vi "generateSignedDecimalFractions.vi"(6 "timeout (10000)":i32=10000, 8 "error in (no error)":errorcluster, 11 "Parameters":T2={"params"={"apiKey"="", "n"=0, "decimalPlaces"=0, "replacement"=TRUE}, "id"=0.0}) -> (0 "error out":errorcluster, 3 "Response":T1={"result"={"random"={"method"="", "hashedApiKey"="", "n"=0, "decimalPlaces"=0, "replacement"=TRUE, "data"=[], "completionTime"="", "serialNumber"=0}, "signature"="", "bitsUsed"=0, "bitsLeft"=0, "requestsLeft"=0, "advisoryDelay"=0}, "id"=0.0} {"result"."random"."data" format="%#_14g"}, 4 "error data":string[](array[string]))   [LabVIEW 2014, in "Random JSON API.lvlib"]
uses:
  Random JSON API.lvlib
  Type Defs/generateDecimalFractionsRequest.ctl
  Type Defs/generateSignedDecimalFractionsResponse.ctl
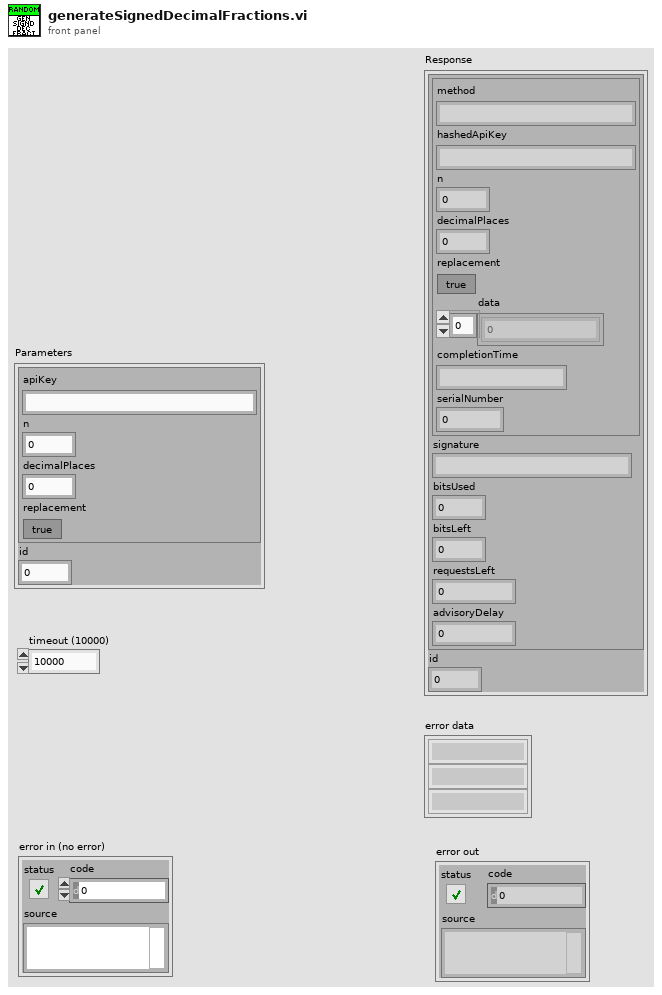
[diagram p1: front panel]
types:
  T1 = typedef "Random JSON API.lvlib/generateSignedDecimalFractionsResponse.ctl" = cluster{"result":cluster{"random":cluster{"method":string, "hashedApiKey":string, "n":i32, "decimalPlaces":i32, "replacement":bool, "data":dbl[], "completionTime":string, "serialNumber":i32}, "signature":string, "bitsUsed":i32, "bitsLeft":i32, "requestsLeft":i32, "advisoryDelay":i32}, "id":dbl}
  T2 = typedef "Random JSON API.lvlib/generateDecimalFractionsRequest.ctl" = cluster{"params":cluster{"apiKey":string, "n":i32, "decimalPlaces":i32, "replacement":bool}, "id":dbl}
  T3 = cluster{"apiKey":string, "n":i32, "decimalPlaces":i32, "replacement":bool}
  T4 = cluster{"jsonrpc":string, "method":string, "params":cluster{"apiKey":string, "n":i32, "decimalPlaces":i32, "replacement":bool}, "id":dbl}
  T5 = cluster{"result cluster":cluster{"completionTime":string, "bitsUsed":i32, "bitsLeft":i32, "requestsLeft":i32, "advisoryDelay":i32}, "method":string, "hashedApiKey":string, "n":i32, "serialNumber":i32, "signature":string}
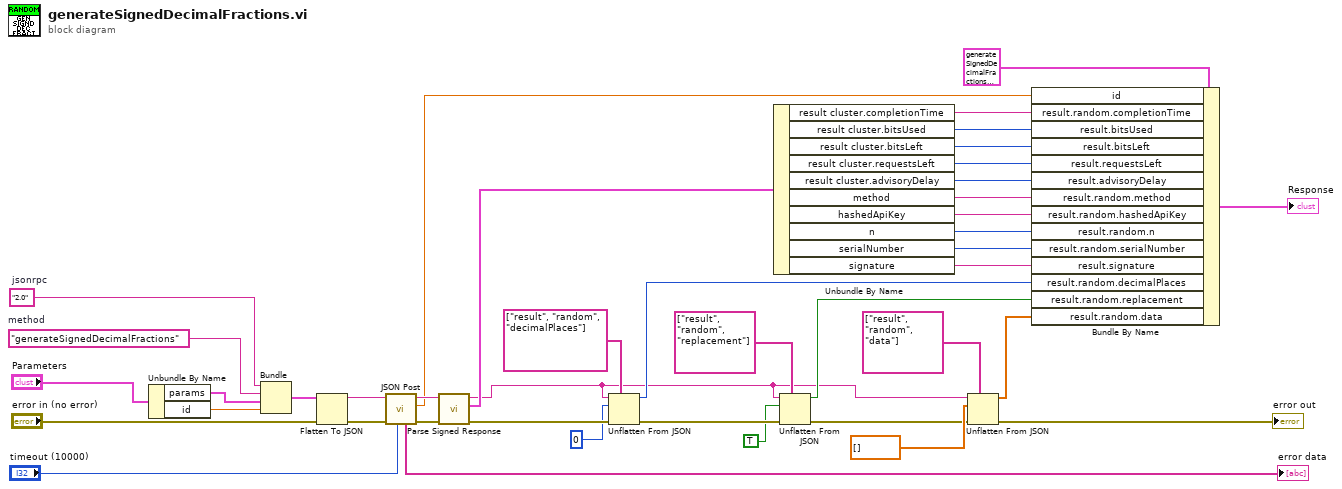
[diagram p0: block diagram]
diagram:
  w27 = "2.0"  # jsonrpc
  w31 = "generateSignedDecimalFractions"  # method
  n1 = Unbundle By Name("Parameters") -> ("params"=w30:T3, "id"=w29:dbl)
  n2 = Bundle("jsonrpc"=w27, "method"=w31, "params"=w30, "id"=w29) -> (w28:T4)  [unwired: 1 in]
  n3 = Flatten To JSON(anything=w28, error in (no error)="error in (no error)") -> (JSON string=w33:string, 11:w34:errorcluster)  [unwired: 1 in]
  n4 = call "JSON Post.vi"("timeout (10000)"="timeout (10000)", "error in (no error)"=w34, "Request JSON String"=w33) -> ("error out"=w40:errorcluster, "id"=w23:dbl, "Response JSON String"=w24:string, "error data"=→"error data":string[])  [unwired: 5 in]
  n5 = call "Parse Signed Response.vi"("error in (no error)"=w40, "body in"=w24) -> ("error out"=w13:errorcluster, "signed result cluster"=w22:T5, "body out"=w6:string)  [unwired: 7 in]
  n6 = Unflatten From JSON(path=string[] ["result", "random", "decimalPlaces"], JSON string=w6, type and defaults=0, error in (no error)=w13) -> (value=w10:i32, error out=w12:errorcluster)  [unwired: 3 in]
  n7 = Unbundle By Name(w22) -> ("result cluster.completionTime"=w39:string, "result cluster.bitsUsed"=w38:i32, "result cluster.bitsLeft"=w37:i32, "result cluster.requestsLeft"=w36:i32, "result cluster.advisoryDelay"=w35:i32, "method"=w5:string, "hashedApiKey"=w4:string, "n"=w3:i32, "serialNumber"=w2:i32, "signature"=w1:string)
  n8 = Unflatten From JSON(path=string[] ["result", "random", "replacement"], JSON string=w6, type and defaults=TRUE, error in (no error)=w12) -> (value=w9:bool, error out=w11:errorcluster)  [unwired: 3 in]
  n9 = Unflatten From JSON(path=string[] ["result", "random", "data"], JSON string=w6, type and defaults=dbl[] [], error in (no error)=w11) -> (value=w16:dbl[], error out=→"error out":errorcluster)  [unwired: 3 in]
  n10 = Bundle By Name(cluster=T1 {"result"={"random"={"method"="", "hashedApiKey"="", "n"=0, "decimalPlaces"=0, "replacement"=TRUE, "data"=[], "completionTime"="", "serialNumber"=0}, "signature"="", "bitsUsed"=0, "bitsLeft"=0, "requestsLeft"=0, "advisoryDelay"=0}, "id"=0.0} ("Response"), "id"=w23, "result.random.completionTime"=w39, "result.bitsUsed"=w38, "result.bitsLeft"=w37, "result.requestsLeft"=w36, "result.advisoryDelay"=w35, "result.random.method"=w5, "result.random.hashedApiKey"=w4, "result.random.n"=w3, "result.random.serialNumber"=w2, "result.signature"=w1, "result.random.decimalPlaces"=w10, "result.random.replacement"=w9, "result.random.data"=w16) -> (→"Response":T1)
